vi "SDCP Receiver and Transmitter - Tx Table Updater - Backup.vi"(5 "Current Cell Position":T2, 7 "Entry position descriptors":cluster{"Start Row":i32, "End Row":i32}[](array[cluster]), 8 "error in (no error)":errorcluster, 10 "Table Control":refnum<vi>, 11 "Tx Table entry cluster array in":T1[](array[typedef])) -> (0 "error out":errorcluster, 3 "Tx Table entry cluster array out":T1[](array[typedef]))   [LabVIEW 2020]
uses:
  <vilib>/Utility/miscctls.llb/LVRowAndColumnTypeDef.ctl
  Typedefs/SDCP SMF Receiver and Transmitter - Transmit Table Element.ctl
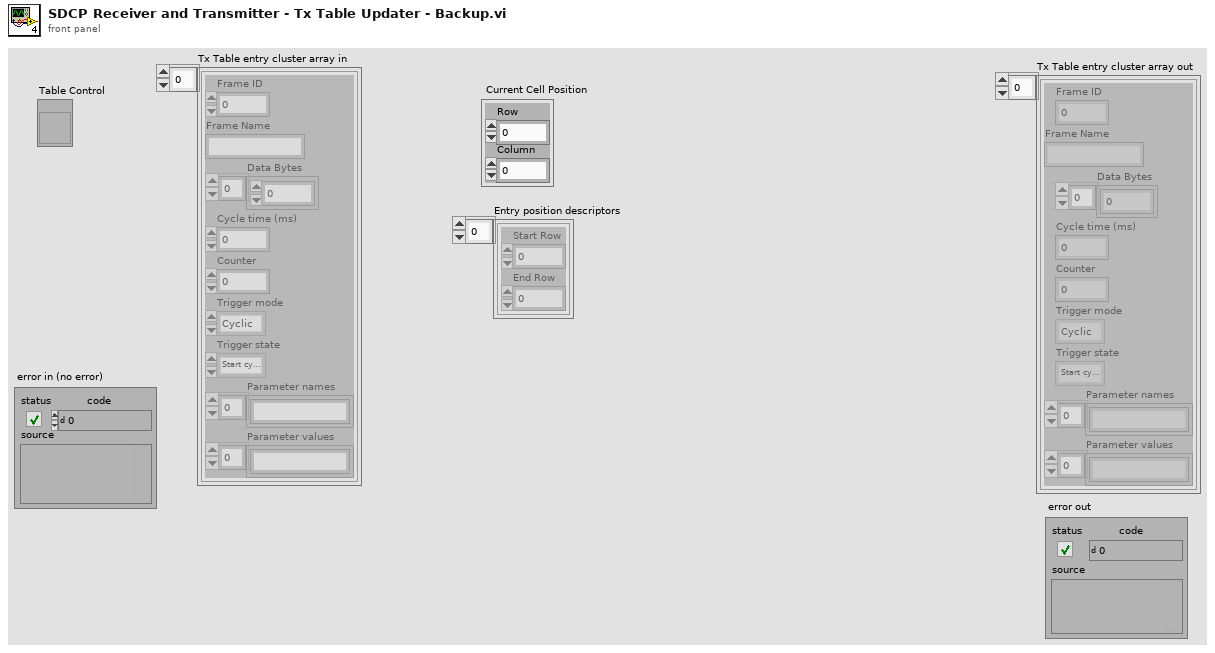
[diagram p1: front panel]
types:
  T1 = typedef "SDCP SMF Receiver and Transmitter - Transmit Table Element.ctl" = cluster{"Frame ID":i32, "Frame Name":string, "Data Bytes":u8[], "Cycle time (ms)":i32, "Counter":i32, "Trigger mode":enum16{"Triggered", "Cyclic"}, "Trigger state":enum16{"Start cyclic trigger", "Stop cyclic trigger", "Start single trigger", "Stop single trigger"}, "Parameter names":string[], "Parameter values":string[]}
  T2 = typedef "LVRowAndColumnTypeDef.ctl" = cluster{"Row":i32, "Column":i32}
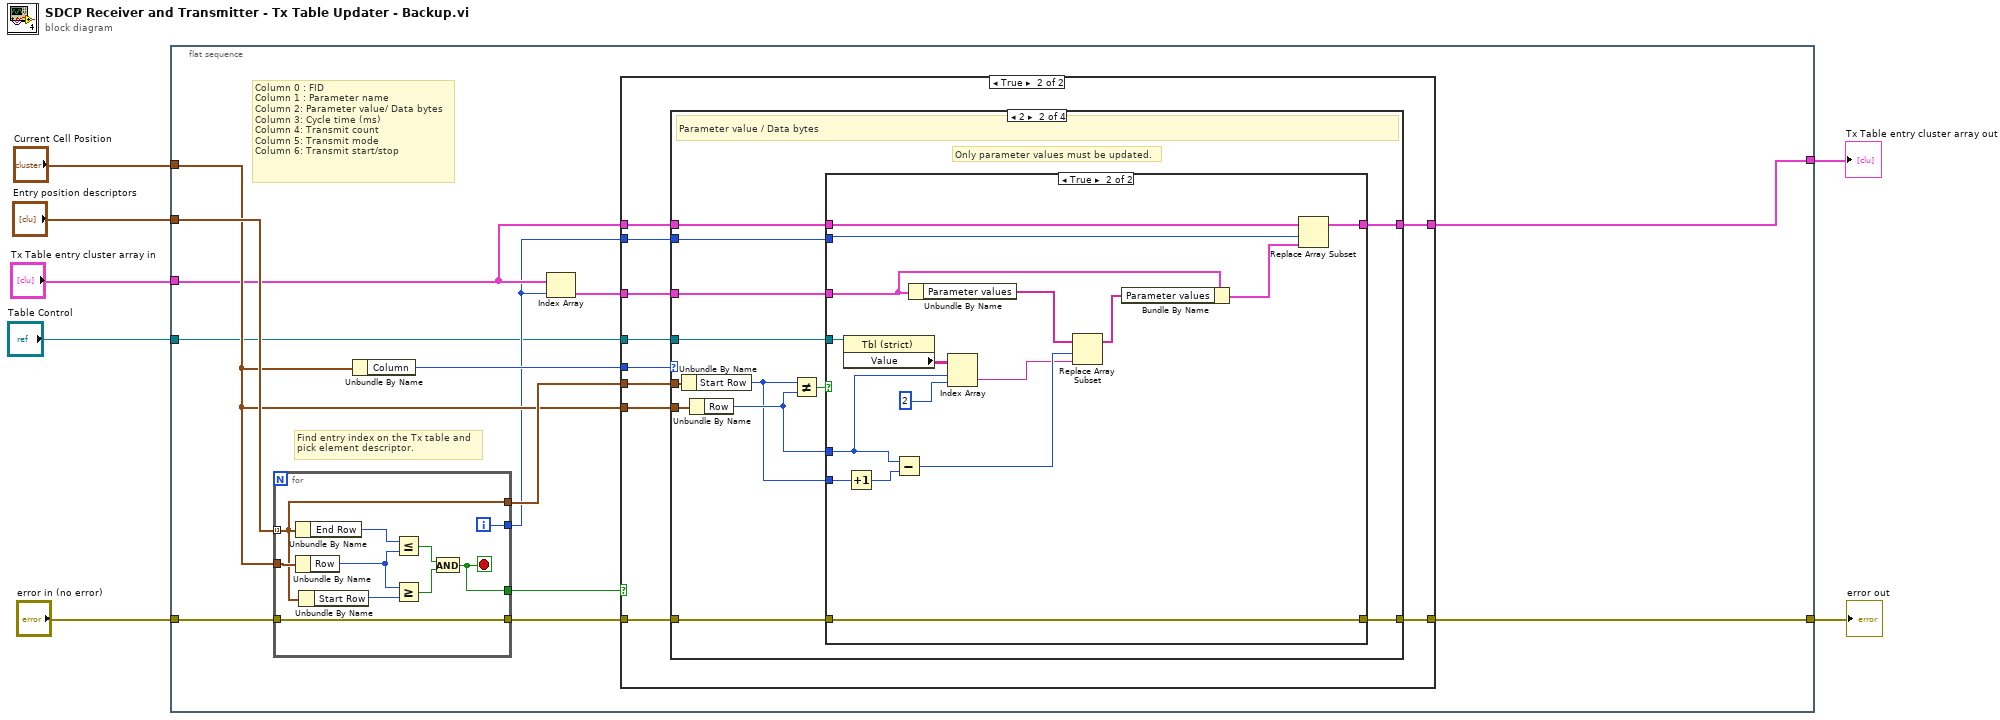
[diagram p0: block diagram]
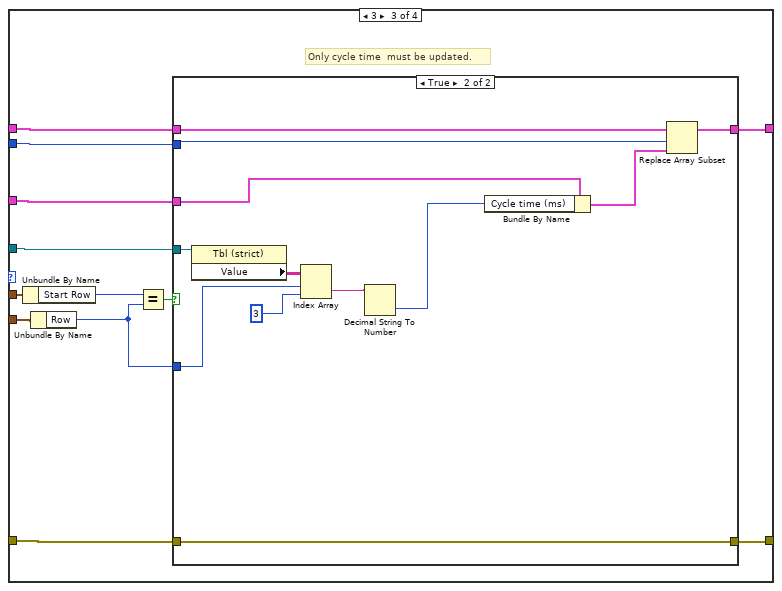
[diagram p5: hidden frame]
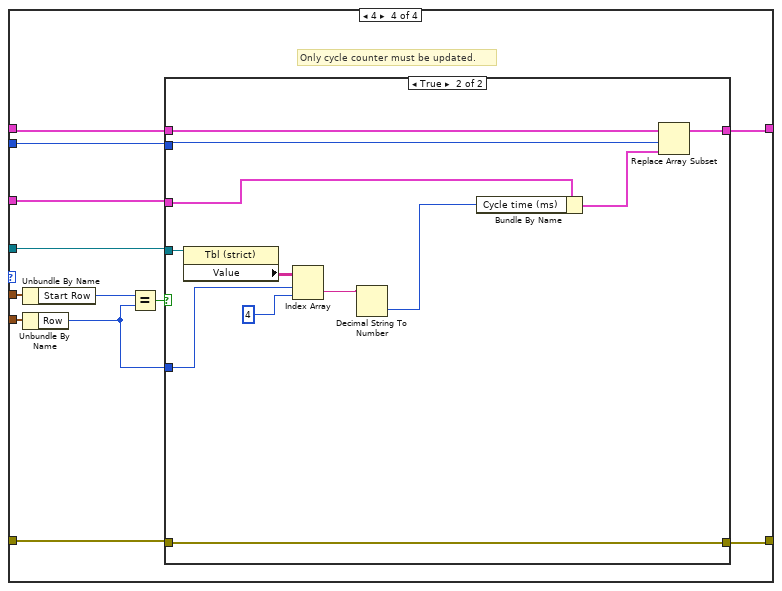
[diagram p7: hidden frame]
diagram:
  n1 = flat-sequence {
    tunnel: "error in (no error)" -> [w19]
    tunnel: "Current Cell Position" -> [w13]
    tunnel: "Entry position descriptors" -> [w20]
    tunnel: "Tx Table entry cluster array in" -> [w12]
    tunnel: "Table Control" -> [w9]
    tunnel: [w15] -> w2
    tunnel: [w11] -> w1
    frame #0 {
      # "Column 0 : FID\nColumn 1 : Parameter name\nColumn 2: Parameter value/ Data bytes\nColumn 3: Cycle time (ms)\nColumn 4: Transmit count\nColumn 5: Transmit mode\nColumn 6: Transmit start/stop"
      # "Find entry index on the Tx table and \npick element descriptor."
      n2 = for {
        tunnel: w20 -> [w118] mode=indexing
        tunnel: w19 -> [w120]
        tunnel: w13 -> [w126]
        tunnel: [w120] -> w18
        tunnel: [w119] -> w10
        tunnel: [w118] -> w14
        tunnel: [w117] -> w8
        i -> [w119]
        stop <- w117 stop-if-true
        n3 = Unbundle By Name(w118) -> ("End Row"=w125:i32)
        n4 = Unbundle By Name(w126) -> ("Row"=w124:i32)
        n5 = Unbundle By Name(w118) -> ("Start Row"=w123:i32)
        n6 = Less Or Equal?(x=w125, y=w124) -> (x <= y?=w122:bool)
        n7 = Greater Or Equal?(x=w124, y=w123) -> (x >= y?=w121:bool)
        n8 = And(x=w122, y=w121) -> (x .and. y?=w117:bool)
      }
      n9 = Unbundle By Name(w13) -> ("Column"=w17:i32)
      n10 = Index Array(array=w12, index=w10) -> (element=w16:T1)
      n11 = case shown="True" w8 {
        tunnel: w18 -> [w21 w32]
        tunnel: w17 -> [_ w31]
        tunnel: w16 -> [_ w30]
        tunnel: [w21 w29] -> w15
        tunnel: w14 -> [_ w28]
        tunnel: w13 -> [_ w27]
        tunnel: w12 -> [w22 w26]
        tunnel: [w22 w25] -> w11
        tunnel: w10 -> [_ w24]
        tunnel: w9 -> [_ w23]
        frame False {
        }
        frame True {
          n12 = case shown="2" w31 {
            tunnel: w32 -> [w34 w43 w67 w97]
            tunnel: w30 -> [_ w37 w71 w95]
            tunnel: [w34 w42 w66 w96] -> w29
            tunnel: w28 -> [_ w46 w69 w92]
            tunnel: w27 -> [_ w45 w68 w91]
            tunnel: w26 -> [w33 w41 w73 w99]
            tunnel: [w33 w40 w65 w98] -> w25
            tunnel: w24 -> [_ w36 w72 w94]
            tunnel: w23 -> [_ w35 w70 w93]
            frame 0, 1, Default {
            }
            frame 2 {
              # "Only parameter values must be updated."
              # "Parameter value / Data bytes"
              n13 = Unbundle By Name(w46) -> ("Start Row"=w38:i32)
              n14 = Unbundle By Name(w45) -> ("Row"=w39:i32)
              n15 = Not Equal?(x=w38, y=w39) -> (x != y?=w44:bool)
              n16 = case shown="True" w44 {
                tunnel: w43 -> [w48 w62]
                tunnel: [w48 w62] -> w42
                tunnel: w41 -> [w47 w57]
                tunnel: [w47 w56] -> w40
                tunnel: w39 -> [_ w51]
                tunnel: w38 -> [_ w64]
                tunnel: w37 -> [_ w59]
                tunnel: w36 -> [_ w55]
                tunnel: w35 -> [_ w53]
                frame False {
                }
                frame True {
                  n17 = property class="Tbl (strict)"(reference=w53) -> ("Value"=w52:string[][])  [unwired: 1 in, 2 out]
                  n18 = Increment(x=w64) -> (x+1=w63:i32)
                  n19 = Subtract(x=w51, y=w63) -> (x-y=w60:i32)
                  n20 = Unbundle By Name(w59) -> ("Parameter values"=w61:string[])
                  n21 = Index Array(array=w52, index (row)=w51, index (col)=2 ("disabled index (col)")) -> (element=w49:string)
                  n22 = Replace Array Subset(array=w61, new element=w49, index=w60) -> (w58:string[])
                  n23 = Bundle By Name(cluster=w59, "Parameter values"=w58) -> (w54:T1)
                  n24 = Replace Array Subset(array=w57, new element=w54, index=w55) -> (w56:T1[])
                }
              }
            }
            frame 3 {
              # "Only cycle time  must be updated."
              n25 = Unbundle By Name(w69) -> ("Start Row"=w74:i32)
              n26 = Unbundle By Name(w68) -> ("Row"=w75:i32)
              n27 = Equal?(x=w74, y=w75) -> (x = y?=w76:bool)
              n28 = case shown="True" w76 {
                tunnel: w67 -> [w78 w90]
                tunnel: [w78 w90] -> w66
                tunnel: w73 -> [w77 w88]
                tunnel: [w77 w87] -> w65
                tunnel: w75 -> [_ w82]
                tunnel: w71 -> [_ w89]
                tunnel: w72 -> [_ w86]
                tunnel: w70 -> [_ w84]
                frame False {
                }
                frame True {
                  n29 = property class="Tbl (strict)"(reference=w84) -> ("Value"=w83:string[][])  [unwired: 1 in, 2 out]
                  n30 = Index Array(array=w83, index (row)=w82, index (col)=3 ("disabled index (col)")) -> (element=w80:string)
                  n31 = Decimal String To Number(string=w80) -> (number=w79:i32)  [unwired: 2 in, 1 out]
                  n32 = Bundle By Name(cluster=w89, "Cycle time (ms)"=w79) -> (w85:T1)
                  n33 = Replace Array Subset(array=w88, new element=w85, index=w86) -> (w87:T1[])
                }
              }
            }
            frame 4 {
              # "Only cycle counter must be updated."
              n34 = Unbundle By Name(w92) -> ("Start Row"=w100:i32)
              n35 = Unbundle By Name(w91) -> ("Row"=w101:i32)
              n36 = Equal?(x=w100, y=w101) -> (x = y?=w102:bool)
              n37 = case shown="True" w102 {
                tunnel: w97 -> [w104 w116]
                tunnel: [w104 w116] -> w96
                tunnel: w99 -> [w103 w114]
                tunnel: [w103 w113] -> w98
                tunnel: w101 -> [_ w108]
                tunnel: w95 -> [_ w115]
                tunnel: w94 -> [_ w112]
                tunnel: w93 -> [_ w110]
                frame False {
                }
                frame True {
                  n38 = property class="Tbl (strict)"(reference=w110) -> ("Value"=w109:string[][])  [unwired: 1 in, 2 out]
                  n39 = Index Array(array=w109, index (row)=w108, index (col)=4 ("disabled index (col)")) -> (element=w106:string)
                  n40 = Decimal String To Number(string=w106) -> (number=w105:i32)  [unwired: 2 in, 1 out]
                  n41 = Bundle By Name(cluster=w115, "Cycle time (ms)"=w105) -> (w111:T1)
                  n42 = Replace Array Subset(array=w114, new element=w111, index=w112) -> (w113:T1[])
                }
              }
            }
          }
        }
      }
    }
  }
  "Tx Table entry cluster array out" <- w1
  "error out" <- w2
